vi "Draw Wheel Axle.vi"(4 "length":dbl, 6 "color (black)":u32(colorbox), 7 "picture info":T1={"picture size"={"Width"=500, "Height"=500}, "pixels per unit"=10.0}, 8 "rotation direction":T3 items=["Clockwise", "Counterclockwise"], 9 "wheel frame angle (rad)":dbl, 10 "global wheel position":cluster{"x":dbl, "y":dbl}, 11 "picture in":picture) -> (3 "picture out":picture)   [LabVIEW 2017, in "NI_Robotics_Steering Picture.lvlib"]
uses:
  <vilib>/robotics/Utilities/Visualization/Steering Visualization/Steering Picture/NI_Robotics_Steering Picture.lvlib
  <vilib>/robotics/Steering/Wheel/Rotation Direction.ctl
  <vilib>/robotics/Utilities/Visualization/Steering Visualization/Steering Picture/Picture Info.ctl
  <vilib>/Utility/miscctls.llb/LVBoundsTypeDef.ctl
  <vilib>/Analysis/coordinate.llb/2D Cartesian Coordinate Rotation (Array).vi
  <vilib>/Analysis/NI_AALPro.lvlib
  <vilib>/robotics/Steering/Wheel/NI_Robotics_Wheel.lvclass
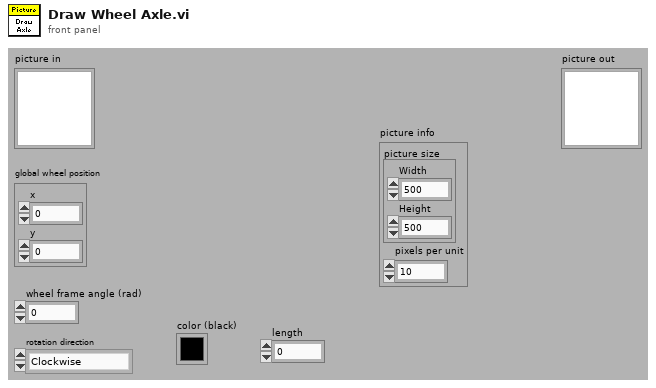
[diagram p1: front panel]
types:
  T1 = typedef "NI_Robotics_Steering Picture.lvlib/Picture Info.ctl" = cluster{"picture size":T2, "pixels per unit":dbl}
  T2 = typedef "LVBoundsTypeDef.ctl" = cluster{"Width":u32, "Height":u32}
  T3 = typedef "NI_Robotics_Wheel.lvclass/Rotation Direction.ctl" = u16
  T4 = cluster{"Width":u16, "Style":enum32{"Solid", "Dash", "Dot", "DashDot", "DashDotDot"}}
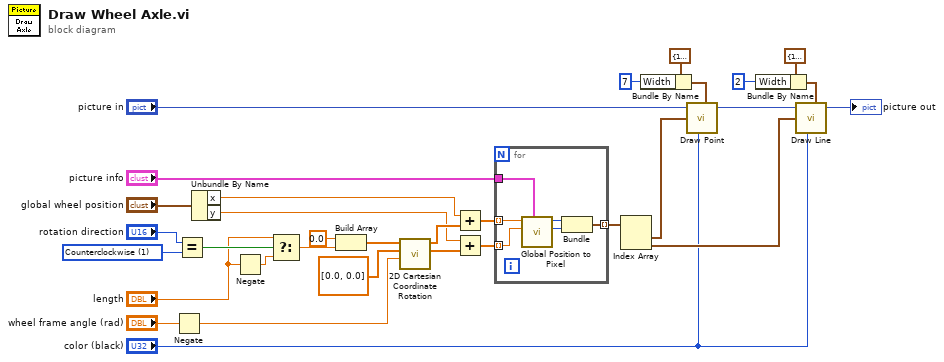
[diagram p0: block diagram]
diagram:
  w10 = T3 1 items=["Clockwise", "Counterclockwise"] ("y")
  n1 = Negate(x="wheel frame angle (rad)") -> (-x=w28:dbl)
  n2 = Equal?(x="rotation direction", y=w10) -> (x = y?=w8:bool)
  n3 = Unbundle By Name("global wheel position") -> ("x"=w25:dbl, "y"=w23:dbl)
  n4 = Negate(x="length") -> (-x=w6:dbl)
  n5 = Select(t="length", s=w8, f=w6) -> (s? t:f=w7:dbl)
  n6 = Build Array(0.0 ("element"), w7) -> (w31:dbl[])
  n7 = call-poly <vilib>:"2D Cartesian Coordinate Rotation.vi"("theta"=w28, "Y"=dbl[] [0.0, 0.0], "X"=w31) -> ("Y Out"=w24:dbl[], "X Out"=w26:dbl[])  [unwired: 6 in, 1 out]
  n8 = Add(x=w25, y=w26) -> (x+y=w22:dbl[])
  n9 = Add(x=w23, y=w24) -> (x+y=w21:dbl[])
  n10 = for {
    tunnel: w22 -> [w38] mode=indexing
    tunnel: w21 -> [w37] mode=indexing
    tunnel: "picture info" -> [w36]
    tunnel: [w33] -> w19 mode=indexing
    n11 = call <vilib>:"Global Position to Pixel.vi"("picture info"=w36, "global y"=w37, "global x"=w38) -> ("pixel y"=w34:i16, "pixel x"=w35:i16)  [unwired: 7 in]
    n12 = Bundle("pixel x"=w35, "pixel y"=w34) -> (w33:cluster{"pixel x":i16, "pixel y":i16})  [unwired: 1 in]
  }
  n13 = Index Array(array=w19) -> (element #1=w18:cluster{"pixel x":i16, "pixel y":i16}, element #2=w13:cluster{"pixel x":i16, "pixel y":i16})  [unwired: 2 in]
  n14 = Bundle By Name(cluster=T4 {"Width"=1, "Style"=enum."Solid"} ("pen"), "Width"=u16 7) -> (w15:T4)
  n15 = call <vilib>:"Draw Point.vi"("picture"="picture in", "point(x,y)"=w18, "color(black)"="color (black)", "pen"=w15) -> ("new picture"=w14:picture)  [unwired: 5 in]
  n16 = Bundle By Name(cluster=T4 {"Width"=1, "Style"=enum."Solid"} ("pen"), "Width"=u16 2) -> (w2:T4)
  n17 = call <vilib>:"Draw Line.vi"("picture"=w14, "end point"=w13, "color(black)"="color (black)", "pen"=w2) -> ("new picture"=→"picture out":picture)  [unwired: 5 in]
